vi "Int Complex To Items.vi"(10 "Numeric Array":cluster{"Numeric Array":i32[]}[](array[cluster])) -> (2 "Items Text":cluster{string[]}[](array[cluster]))   [LabVIEW 2024]
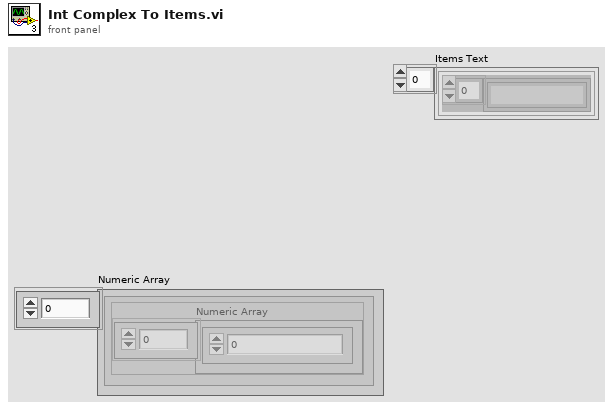
[diagram p1: front panel]
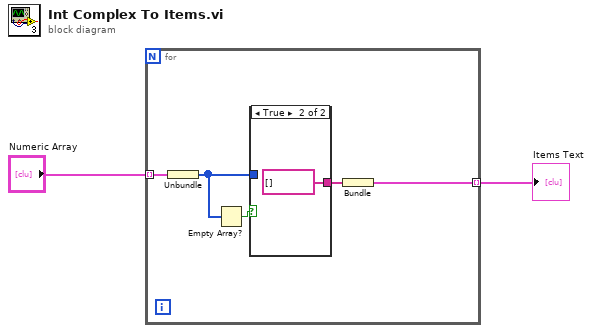
[diagram p0: block diagram]
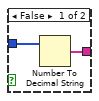
[diagram p2: hidden frame]
diagram:
  n1 = for {
    tunnel: "Numeric Array" -> [w7] mode=indexing
    tunnel: [w5] -> w1 mode=indexing
    n2 = Unbundle(w7) -> ("Numeric Array"=w4:i32[])
    n3 = Empty Array?(array=w4) -> (empty?=w3:bool)
    n4 = case shown="True" w3 {
      tunnel: [w9 string[] []] -> w6
      tunnel: w4 -> [w8 _]
      frame False {
        n5 = Number To Decimal String(number=w8) -> (decimal integer string=w9:string[])  [unwired: 1 in]
      }
      frame True {
      }
    }
    n6 = Bundle(w6) -> (w5:cluster{string[]})  [unwired: 1 in]
  }
  "Items Text" <- w1
